vi "Day 12 Puzzle 1 Another angle.vi"(11 "Path":path) -> ()   [LabVIEW 2021]
uses:
  <vilib>/Utility/file.llb/Read Delimited Spreadsheet (string).vi
panel:
  out "x .or. y?":bool[](array[boolean])
  out "number":u32
  out "appended array 2":i32[](array[numeric])
  out "max index(es)":i32
  out "appended array":i32[](array[numeric])
  out "x+1":i32
  out "size(s)":i32[](array[numeric])
  out "Array":i32[][](array[numeric])
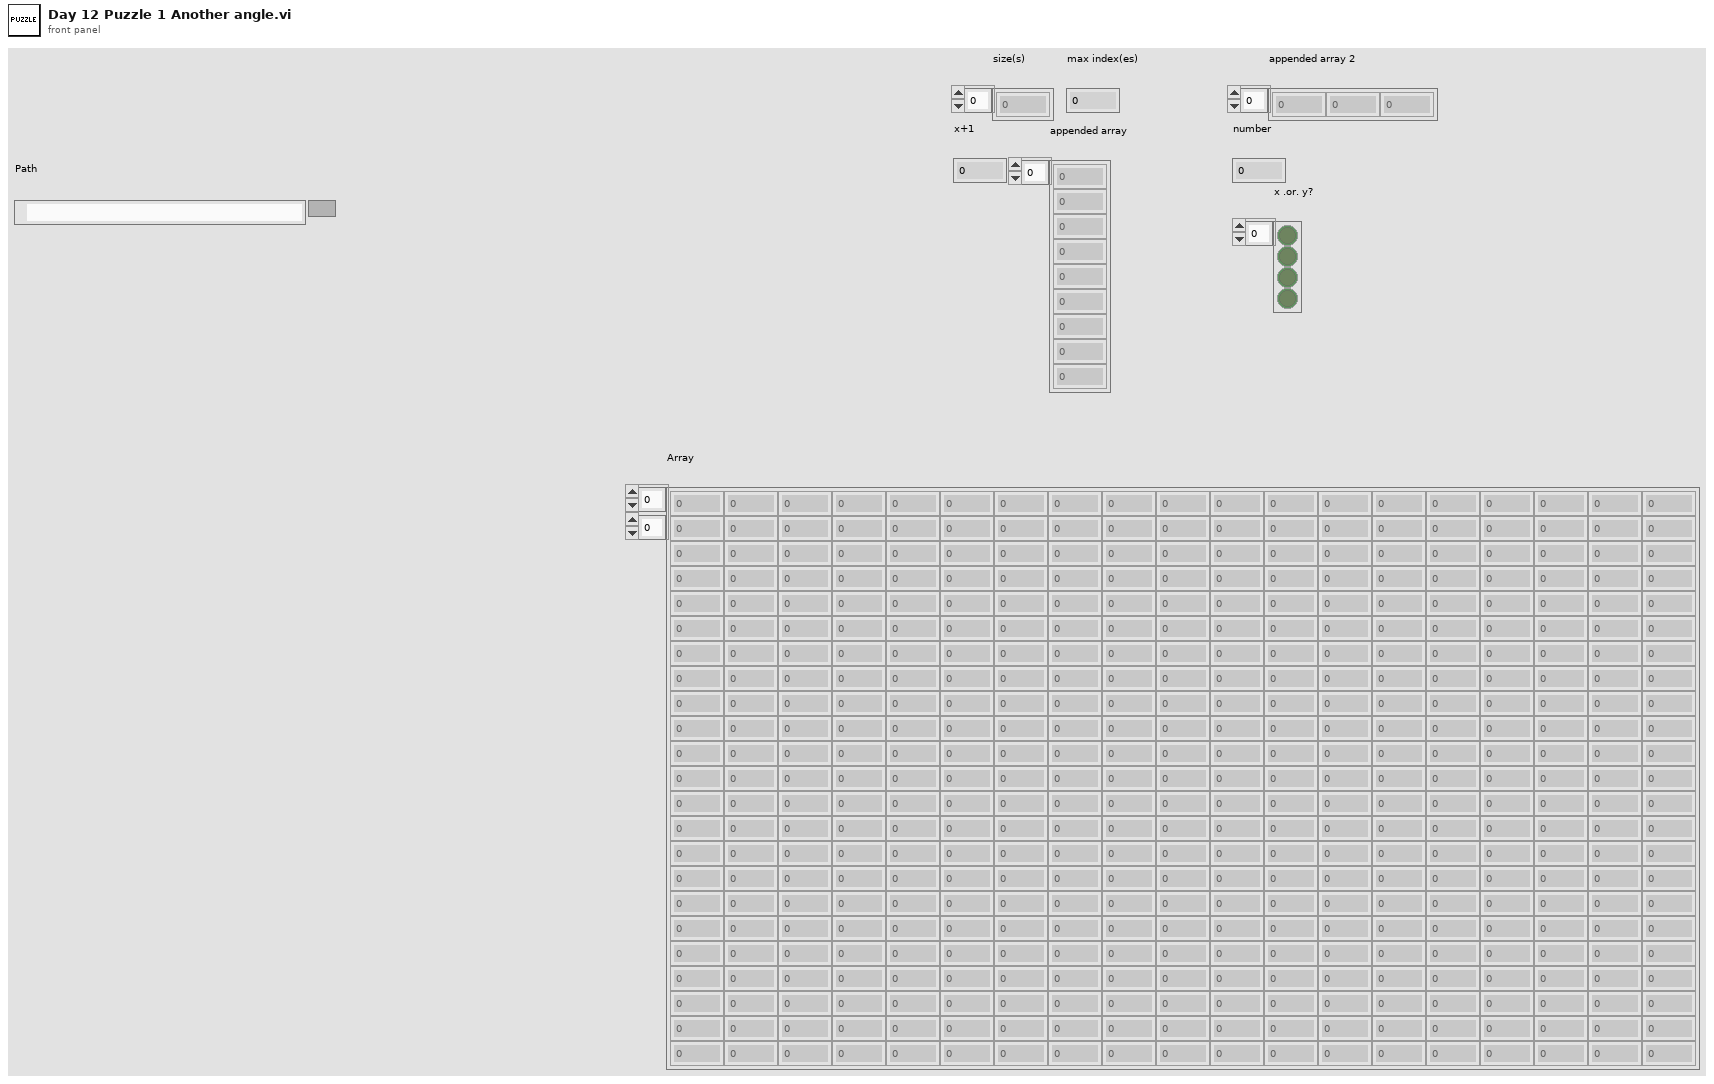
[diagram p1: front panel]
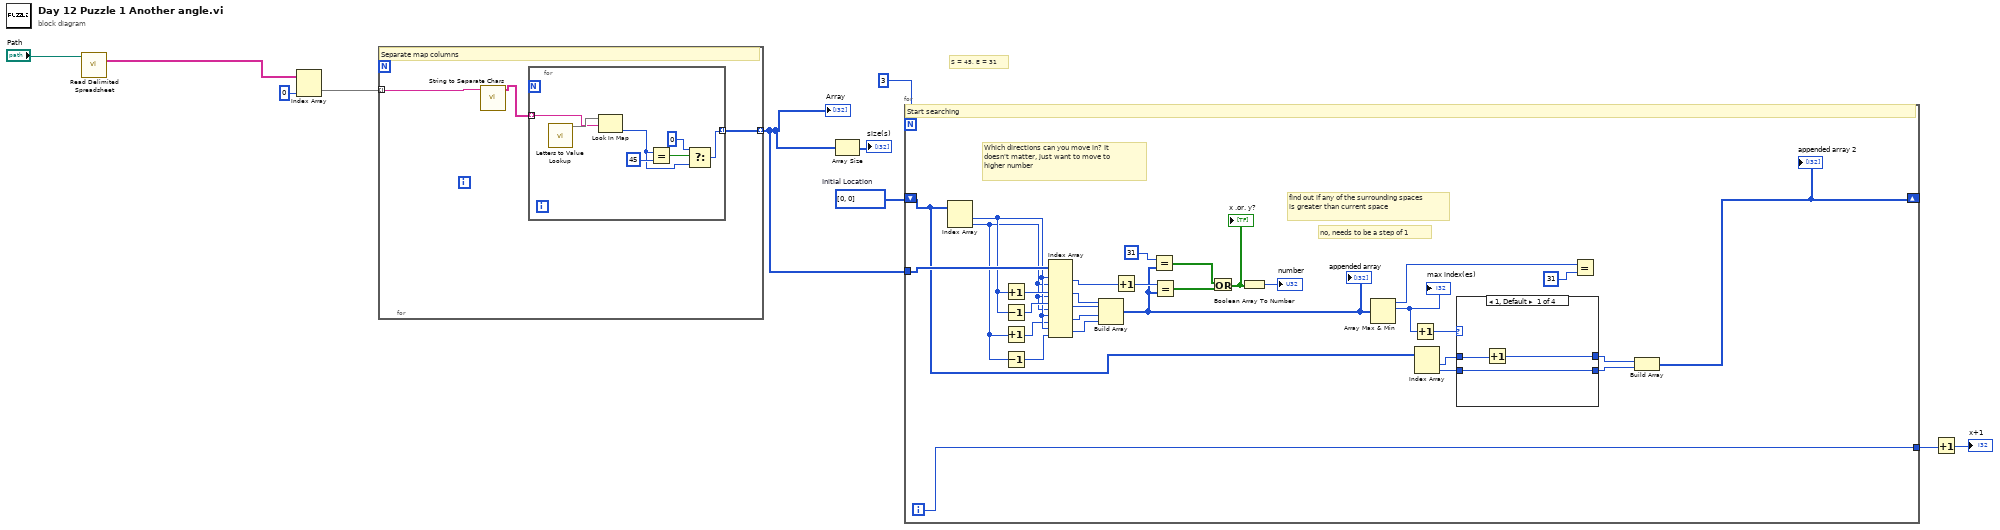
[diagram p0: block diagram]
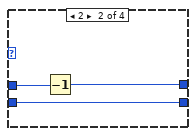
[diagram p2: hidden frame]
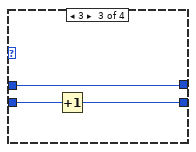
[diagram p3: hidden frame]
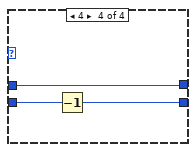
[diagram p4: hidden frame]
diagram:
  w5 = i32[] [0, 0]  # Initial Location
  # "S = 45, E = 31"
  n1 = call-poly <vilib>:"Read Delimited Spreadsheet.vi"("file path (dialog if empty)"="Path") -> ("all rows"=w9:string[][])  [unwired: 9 in, 5 out]
  n2 = Index Array(array=w9, index (col)=0 ("disabled index (col)")) -> (element=w7:string[])  [unwired: 1 in]
  n3 = for {
    tunnel: w7 -> [w13] mode=indexing
    tunnel: [w11] -> w1 mode=indexing
    # "Separate map columns"
    n4 = call "String to Separate Chars.vi"("String"=w13) -> ("Array"=w12:string[])  [unwired: 10 in]
    n5 = for {
      tunnel: w12 -> [w19] mode=indexing
      tunnel: [w14] -> w11 mode=indexing
      n6 = call "Letters to Value Lookup.vi"() -> ("map in"=w20:map{string, i32})  [unwired: 11 in]
      n7 = Look In Map(map=w20, key=w19) -> (value=w16:i32)  [unwired: 1 in, 1 out]
      n8 = Equal?(x=w16, y=45) -> (x = y?=w17:bool)
      n9 = Select(t=0, s=w17, f=w16) -> (s? t:f=w14:i32)
    }
  }
  "Array" <- w1
  n10 = Array Size(array=w1) -> (size(s)=→"size(s)":i32[])
  n11 = for {
    N: 3 -> [_]
    tunnel: w1 -> [w50]
    shift-right: [w32] -> _
    shift-left: w5 -> [w38]
    tunnel: [w29] -> w4
    i -> [w29]
    # "no, needs to be a step of 1"
    # "find out if any of the surrounding spaces is greater than current space"
    # "Which directions can you move in? It doesn't matter, just want to move to higher number"
    # "Start searching"
    n12 = Index Array(array=w38) -> (element #1=w47:i32, element #2=w45:i32)  [unwired: 2 in]
    n13 = Increment(x=w47) -> (x+1=w49:i32)
    n14 = Decrement(x=w47) -> (x-1=w48:i32)
    n15 = Increment(x=w45) -> (x+1=w46:i32)
    n16 = Decrement(x=w45) -> (x-1=w44:i32)
    n17 = Index Array(array=w50, index (row) #1=w47, index (col) #1=w45, index (row) #2=w49, index (col) #2=w45, index (row) #3=w48, index (col) #3=w45, index (row) #4=w47, index (col) #4=w46, index (row) #5=w47, index (col) #5=w44) -> (element #1=w28:i32, element #2=w43:i32, element #3=w42:i32, element #4=w41:i32, element #5=w40:i32)
    n18 = Build Array(w43, w42, w41, w40) -> (w25:i32[])
    "appended array" <- w25
    n19 = Increment(x=w28) -> (x+1=w27:i32)
    n20 = Equal?(x=31 ("element"), y=w25) -> (x = y?=w24:bool[])
    n21 = Equal?(x=w27, y=w25) -> (x = y?=w23:bool[])
    n22 = Or(x=w24, y=w23) -> (x .or. y?=w22:bool[])
    "x .or. y?" <- w22
    n23 = Boolean Array To Number(Boolean array=w22) -> (number=→"number":u32)
    n24 = Array Max & Min(array=w25) -> (max value=w31:i32, max index (indices)=w39:i32)  [unwired: 2 out]
    "max index(es)" <- w39
    n25 = Increment(x=w39) -> (x+1=w33:i32)
    n26 = Index Array(array=w38) -> (element #1=w37:i32, element #2=w36:i32)  [unwired: 2 in]
    n27 = case shown="1, Default" w33 {
      tunnel: w37 -> [w53 w56 w59 w62]
      tunnel: w36 -> [w51 w54 w58 w61]
      tunnel: [w52 w55 w59 w62] -> w35
      tunnel: [w51 w54 w57 w60] -> w34
      frame 1, Default {
        n28 = Increment(x=w53) -> (x+1=w52:i32)
      }
      frame 2 {
        n29 = Decrement(x=w56) -> (x-1=w55:i32)
      }
      frame 3 {
        n30 = Increment(x=w58) -> (x+1=w57:i32)
      }
      frame 4 {
        n31 = Decrement(x=w61) -> (x-1=w60:i32)
      }
    }
    n32 = Equal?(x=w31, y=31) -> ()  [unwired: 1 out]
    n33 = Build Array(w35, w34) -> (w32:i32[])
    "appended array 2" <- w32
  }
  n34 = Increment(x=w4) -> (x+1=→"x+1":i32)
